vi "EnterPW.vi"(7 "error in":errorcluster) -> (0 "error out":errorcluster, 2 "Prod":bool caption="Product", 3 "Tech":bool, 9 "YN Msg 2":string)   [LabVIEW 2017]
panel:
  in  "YN Msg 3":string
  in  "\"Enter\"":bool
  out "yn":bool caption="YN1"
  in  "YN2":bool
  # "Enter Password"
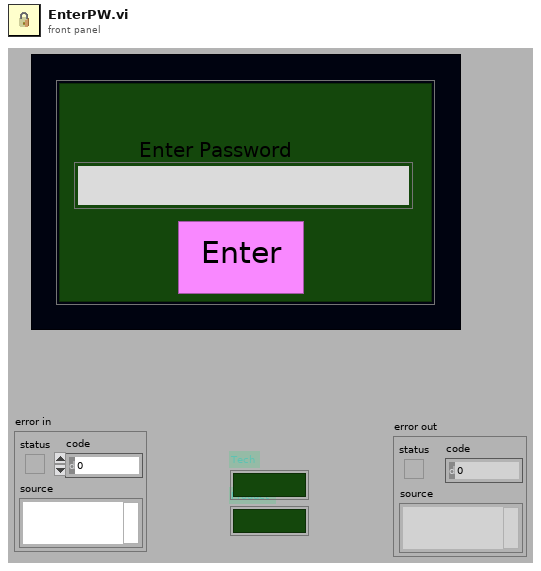
[diagram p1: front panel]
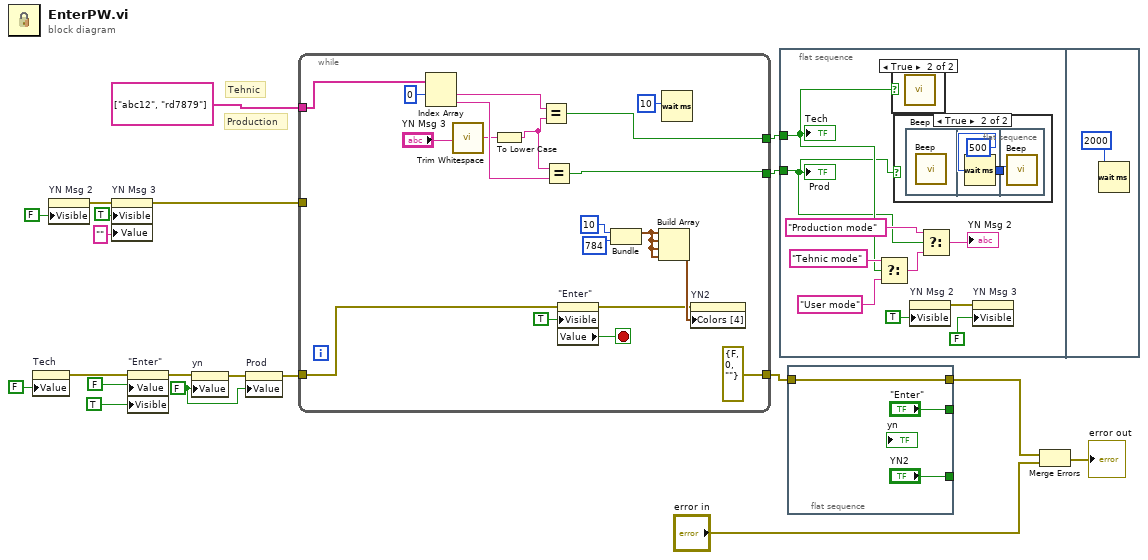
[diagram p0: block diagram]
diagram:
  w11 = FALSE ("Tech")
  # "Production"
  # "Tehnic"
  n1 = property on="Tech" class="Bool (strict)"("Value"=FALSE ("Tech")) -> (error out=w10:errorcluster)  [unwired: 2 in, 1 out]
  n2 = property on="YN Msg 2" class="Str"("Visible"=FALSE) -> (error out=w4:errorcluster)  [unwired: 2 in, 1 out]
  n3 = property on="YN Msg 3" class="Str"(error in=w4, "Visible"=TRUE, "Value"="" ("YN Msg 3")) -> (error out=w5:errorcluster)  [unwired: 1 in, 1 out]
  n4 = property on="\"Enter\"" class="Bool (strict)"(error in=w10, "Value"=FALSE ("\"YES\""), "Visible"=TRUE ("\"YES\"")) -> (error out=w14:errorcluster)  [unwired: 1 in, 1 out]
  n5 = property on="yn" class="Bool (strict)"(error in=w14, "Value"=w11) -> (error out=w13:errorcluster)  [unwired: 1 in, 1 out]
  n6 = property on="Prod" class="Bool (strict)"(error in=w13, "Value"=w11) -> (error out=w12:errorcluster)  [unwired: 1 in, 1 out]
  n7 = while {
    tunnel: w12 -> [w36]
    tunnel: [errorcluster {"status"=FALSE, "code"=0, "source"=""} ("error out")] -> w20
    tunnel: string[] ["abc12", "rd7879"] -> [w32]
    tunnel: [w25] -> w6
    tunnel: [w24] -> w7
    tunnel: w5 -> [_]
    stop <- w27 stop-if-true
    n8 = Index Array(array=w32, index #1=0 ("index")) -> (element #1=w30:string, element #2=w28:string)  [unwired: 1 in]
    n9 = call <vilib>:"Trim Whitespace.vi"("string"="YN Msg 3") -> ("trimmed string"=w26:string)  [unwired: 1 in]
    n10 = To Lower Case(string=w26) -> (all lower case string=w29:string)
    n11 = Equal?(x=w30, y=w29) -> (x = y?=w25:bool)
    n12 = Equal?(x=w29, y=w28) -> (x = y?=w24:bool)
    n13 = property on="\"Enter\"" class="Bool (strict)"(error in=w36, "Visible"=TRUE) -> (error out=w34:errorcluster, "Value"=w27:bool)  [unwired: 1 in, 1 out]
    n14 = Bundle(10, 784) -> (w38:cluster{i32, i32})  [unwired: 1 in]
    n15 = Build Array(w38, w38, w38, w38) -> (w37:cluster{i32, i32}[])
    n16 = Wait (ms)(milliseconds to wait=10) -> ()  [unwired: 1 out]
    n17 = property on="YN2" class="Bool (strict)"(error in=w34, "Colors [4]"=w37) -> ()  [unwired: 1 in, 2 out]
  }
  n18 = flat-sequence {
    tunnel: w7 -> [w40]
    tunnel: w6 -> [w41]
    frame #0 {
      n19 = Select(t="Tehnic mode" ("YN Msg 2"), s=w41, f="User mode" ("YN Msg 2")) -> (s? t:f=w48:string)
      n20 = case shown="True" w41 {
        frame False {
        }
        frame True {
          n21 = call <vilib>:"Beep.vi"() -> ()  [unwired: 12 in]
        }
      }
      n22 = case shown="True" w40 {
        frame False {
        }
        frame True {
          n23 = flat-sequence {
            tunnel: [w52] -> w50
            tunnel: w50 -> [w53]
            frame #0 {
              n24 = call <vilib>:"Beep.vi"() -> ()  [unwired: 12 in]
            }
            frame #1 {
              n25 = Wait (ms)(milliseconds to wait=u32 500) -> (millisecond timer value=w52:u32)
            }
            frame #2 {
              n26 = call <vilib>:"Beep.vi"("duration (msec)"=w53) -> ()  [unwired: 11 in]
            }
          }
        }
      }
      n27 = property on="YN Msg 2" class="Str"("Visible"=TRUE) -> (error out=w43:errorcluster)  [unwired: 2 in, 1 out]
      n28 = Select(t="Production mode" ("YN Msg 2"), s=w40, f=w48) -> (s? t:f=→"YN Msg 2":string)
      n29 = property on="YN Msg 3" class="Str"(error in=w43, "Visible"=FALSE) -> ()  [unwired: 1 in, 2 out]
      "Prod" <- w40
      "Tech" <- w41
    }
    frame #1 {
      n30 = Wait (ms)(milliseconds to wait=u32 2000) -> ()  [unwired: 1 out]
    }
  }
  n31 = flat-sequence {
    tunnel: w20 -> [w55]
    tunnel: [w55] -> w17
    tunnel: ["\"Enter\""] -> _
    tunnel: ["YN2"] -> _
    frame #0 {
    }
  }
  n32 = Merge Errors(w17, "error in") -> (→"error out":errorcluster)
